vi "superhetero.vi"() -> ()   [LabVIEW 2009]
uses:
  <vilib>/Analysis/NI_AALBase.lvlib
panel:
  in  "増幅率":dbl
  in  "雑音振幅":dbl
  in  "Q2":dbl
  in  "Q1":dbl
  out "歪み率":dbl
  out "出力":cluster{dbl[], dbl[]}(graph) caption="XYグラフ"
  out "送信波":cluster{dbl[], dbl[]}(graph)
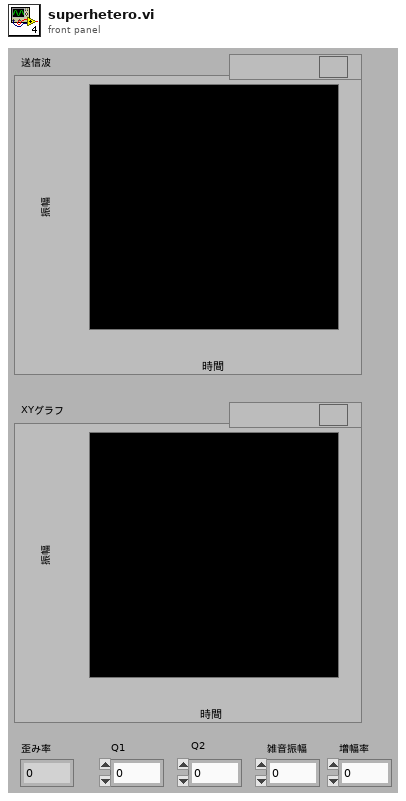
[diagram p1: front panel]
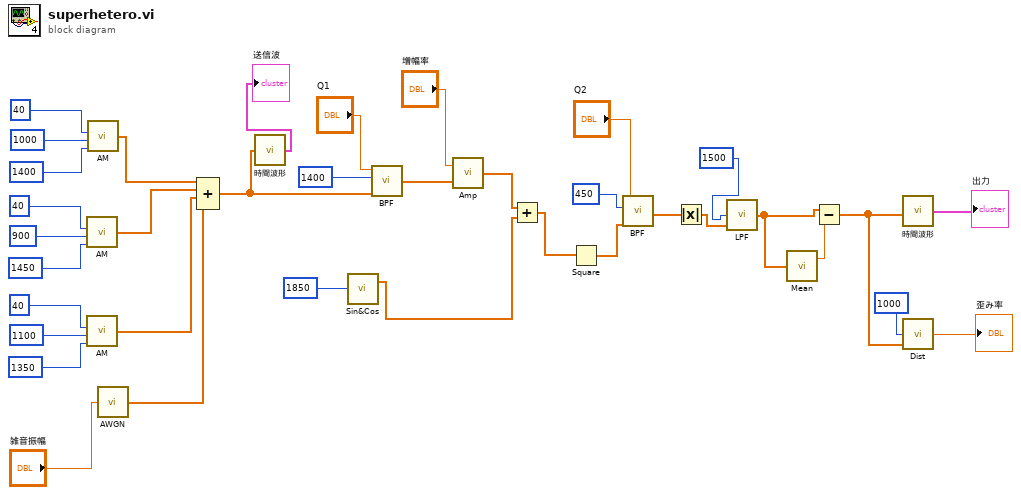
[diagram p0: block diagram]
diagram:
  n1 = call "AM.vi"("変調度 [%]"=40, "変調周波数 [Hz]"=900, "搬送波周波数 [kHz]"=1450) -> ("変調波"=w26:dbl[])  [unwired: 2 in]
  n2 = call "AM.vi"("変調度 [%]"=40, "変調周波数 [Hz]"=1100, "搬送波周波数 [kHz]"=1350) -> ("変調波"=w25:dbl[])  [unwired: 2 in]
  n3 = call "AM.vi"("変調度 [%]"=40, "変調周波数 [Hz]"=1000, "搬送波周波数 [kHz]"=1400) -> ("変調波"=w27:dbl[])  [unwired: 2 in]
  n4 = call "AWGN.vi"("振幅値"="雑音振幅") -> ("出力"=w24:dbl[])
  n5 = Compound Arithmetic op=ADD(w27, w26, w25, w24) -> (w22:dbl[])
  n6 = call "時間波形.vi"("入力"=w22) -> ("時間波形"=→"送信波":cluster{dbl[], dbl[]})
  n7 = call "Sin&Cos.vi"("周波数[kHz]"=1850) -> ("sin"=w7:dbl[])  [unwired: 1 out]
  n8 = call "BPF.vi"("X"=w22, "中心周波数 [kHz]"=1400, "Q"="Q1") -> ("BPF出力"=w9:dbl[])  [unwired: 1 in]
  n9 = call "Amp.vi"("入力"=w9, "増幅率"="増幅率") -> ("出力"=w8:dbl[])
  n10 = Add(x=w8, y=w7) -> (x+y=w6:dbl[])
  n11 = Square(x=w6) -> (x^2=w5:dbl[])
  n12 = call "BPF.vi"("X"=w5, "中心周波数 [kHz]"=450, "Q"="Q2") -> ("BPF出力"=w16:dbl[])  [unwired: 1 in]
  n13 = Absolute Value(x=w16) -> (abs(x)=w15:dbl[])
  n14 = call "LPF.vi"("入力"=w15, "カットオフ周波数 [Hz]"=1500) -> ("LPF出力"=w13:dbl[])  [unwired: 1 in]
  n15 = call <vilib>:"Mean.vi"("X"=w13) -> ("mean"=w14:dbl)  [unwired: 1 out]
  n16 = Subtract(x=w13, y=w14) -> (x-y=w12:dbl[])
  n17 = call "時間波形.vi"("入力"=w12) -> ("時間波形"=→"出力":cluster{dbl[], dbl[]})
  n18 = call "Dist.vi"("入力"=w12, "基本周波数 [Hz]"=1000) -> ("ひずみ率"=→"歪み率":dbl)  [unwired: 1 in]
